vi "Device Files v1.vi"(10 "Rows":i32=80, 11 "Mask file path":path=path "C:/Documents and Settings/sjguest/Desktop/PVIV LV/Excel Files For Device Runs/All Devices.xls") -> (1 "Mask Name":string, 2 "size(s)":i32, 3 "Array of Cell Clusters":T2(array[cluster]), 4 "Alignment Spacing":cluster{"xintv":dbl, "yintv":dbl})   [LabVIEW 2012]
uses:
  <vilib>/imath/engines/lvmath2/RunTimeEngine/ErrorHandling/NIMS_Finalize Error.vi
  <vilib>/imath/engines/lvmath2/RunTimeEngine/NodeEndStatement/NIMS_NodeEndStatement_Output.vi
  <instcachedir>/0/NIMS_NodeEndStatement_Output_53EC0D466D134D7ABD903AC30B43404B.lvgen/NIMS_NodeEndStatement_Output_53EC0D466D134D7ABD903AC30B43404B_001.vi
  <vilib>/imath/engines/lvmath2/RunTimeEngine/BuiltInFunctions/sets_unique/NIMS_sets_unique(GV).vi
  <instcachedir>/0/NIMS_sets_unique(GV)_31CBCD1A87194FEB9DEFC0CB30627D6C.lvgen/NIMS_sets_unique(GV)_31CBCD1A87194FEB9DEFC0CB30627D6C_001.vi
  <vilib>/imath/engines/lvmath2/RunTimeEngine/BuiltInFunctions/length/NIMS_length(GV).vi
  <instcachedir>/0/NIMS_length(GV)_08A3D13377FD4E4B96F5795FBF3698FA.lvgen/NIMS_length(GV)_08A3D13377FD4E4B96F5795FBF3698FA_000.vi
  <vilib>/imath/engines/lvmath2/RunTimeEngine/BuiltInFunctions/abs/NIMS_abs(signed).vi
  <instcachedir>/0/NIMS_abs(signed)_C4FCB8E6058B49B797C7C8D53CA5F6EC.lvgen/NIMS_abs(signed)_C4FCB8E6058B49B797C7C8D53CA5F6EC_000.vi
  <vilib>/regexp/Match Regular Expression.xnode
panel:
  in  "Cell Info Cluster 2":T1={"Cell Name"="10000_150_06", "X-coord"=8850.0, "Y-coord"=8250.0, "Area"=99830016.0, "Grid Shadowing"=99830016.0, "Xdim"=99830016.0, "Ydim"=99830016.0, "Mesa Area"=0.0}
  out "yintv":dbl
  out "xintv":dbl
  out "data":dbl[][](array[numeric])
  out "Loop Count":i32
  out "selection":bool
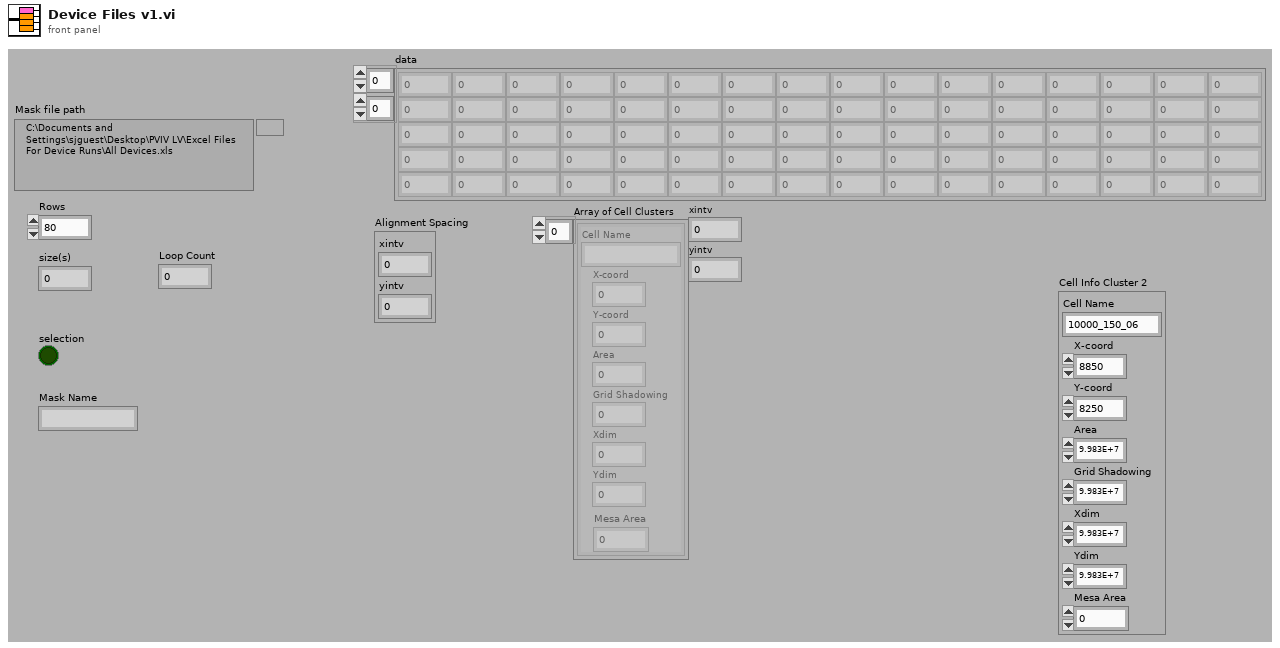
[diagram p1: front panel]
types:
  T1 = cluster{"Cell Name":string, "X-coord":dbl, "Y-coord":dbl, "Area":dbl, "Grid Shadowing":dbl, "Xdim":dbl, "Ydim":dbl, "Mesa Area":dbl}
  T2 = cluster{"Cell Name":string, "X-coord":dbl, "Y-coord":dbl, "Area":dbl, "Grid Shadowing":dbl, "Xdim":dbl, "Ydim":dbl, "Mesa Area":dbl}[]
  T3 = cluster{"disabled index (col)":i32, "disabled index (col)":i32}
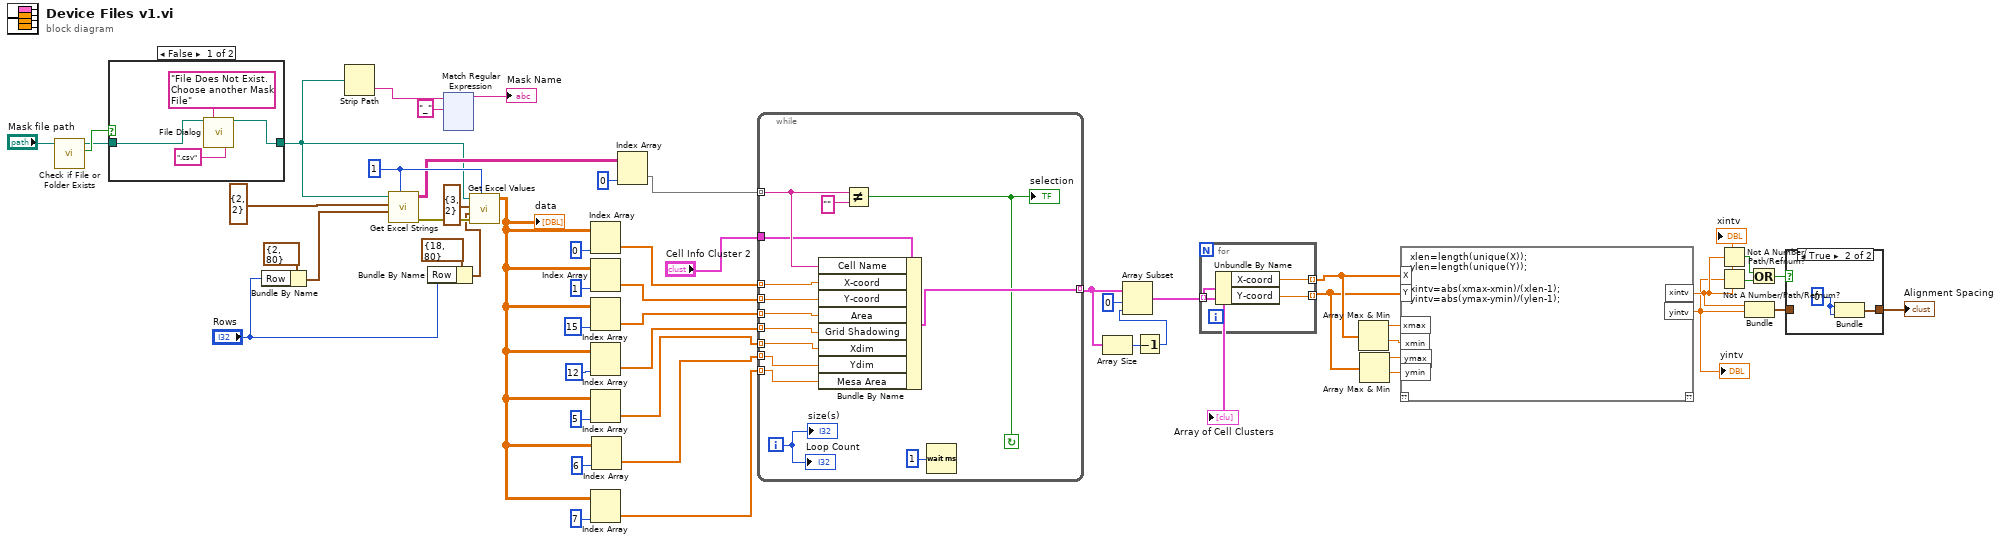
[diagram p0: block diagram]
diagram:
  w46 = 1 ("Sheet")
  n1 = call <vilib>:"Check if File or Folder Exists.vi"("path"="Mask file path") -> ("file or folder exists?"=w24:bool, "dup path"=w22:path)  [unwired: 8 in, 1 out]
  n2 = case shown="False" w24 {
    tunnel: [w56 w58] -> w23
    tunnel: w22 -> [w57 w58]
    frame False {
      n3 = call "File Dialog"("start path"=w57, "prompt"="File Does Not Exist.  Choose another Mask File", "pattern label"=".csv" ("pattern (all files)")) -> ("selected path"=w56:path)  [unwired: 9 in, 3 out]
    }
    frame True {
    }
  }
  n4 = Bundle By Name(cluster=cluster{"Column":i32, "Row":i32} {"Column"=2, "Row"=80} ("End"), "Row"="Rows") -> (w39:cluster{"Column":i32, "Row":i32})
  n5 = Strip Path(path=w23) -> (name=w28:string)  [unwired: 1 out]
  n6 = call "Get Excel Strings.vi"("Sheet"=w46, "End"=w39, "Start"=cluster{"Column":i32, "Row":i32} {"Column"=2, "Row"=2}, "path"=w23) -> ("error out"=w45:errorcluster, "data"=w42:string[][])  [unwired: 1 in, 5 out]
  n7 = Bundle By Name(cluster=cluster{"Column":i32, "Row":i32} {"Column"=18, "Row"=80} ("End"), "Row"="Rows") -> (w37:cluster{"Column":i32, "Row":i32})
  n8 = xnode "Match Regular Expression"("input string"=w28, "regular expression"="_") -> ("before match"=→"Mask Name":string)  [unwired: 2 in, 6 out]
  n9 = call "Get Excel Values.vi"("Sheet"=w46, "error in (no error)"=w45, "End"=w37, "Start"=cluster{"Column":i32, "Row":i32} {"Column"=3, "Row"=2}, "path"=w23) -> ("data"=w3:dbl[][])  [unwired: 6 out]
  "data" <- w3
  n10 = Index Array(array=w3, index (col)=0 ("disabled index (col)")) -> (element=w49:dbl[])  [unwired: 1 in]
  n11 = Index Array(array=w3, index (col)=1 ("disabled index (col)")) -> (element=w48:dbl[])  [unwired: 1 in]
  n12 = Index Array(array=w3, index (col)=15 ("disabled index (col)")) -> (element=w47:dbl[])  [unwired: 1 in]
  n13 = Index Array(array=w3, index (col)=12 ("disabled index (col)")) -> (element=w33:dbl[])  [unwired: 1 in]
  n14 = Index Array(array=w3, index (col)=5 ("disabled index (col)")) -> (element=w12:dbl[])  [unwired: 1 in]
  n15 = Index Array(array=w3, index (col)=7 ("disabled index (col)")) -> (element=w2:dbl[])  [unwired: 1 in]
  n16 = Index Array(array=w3, index (col)=6 ("disabled index (col)")) -> (element=w11:dbl[])  [unwired: 1 in]
  n17 = Index Array(array=w42, index (col)=0 ("disabled index (col)")) -> (element=w53:string[])  [unwired: 1 in]
  n18 = while {
    tunnel: w53 -> [w67] mode=indexing
    tunnel: w49 -> [w70] mode=indexing
    tunnel: w48 -> [w69] mode=indexing
    tunnel: w47 -> [w68] mode=indexing
    tunnel: "Cell Info Cluster 2" -> [w66]
    tunnel: [w64] -> w25 mode=indexing
    tunnel: w33 -> [w65] mode=indexing
    tunnel: w12 -> [w61] mode=indexing
    tunnel: w11 -> [w60] mode=indexing
    tunnel: w2 -> [w59] mode=indexing
    i -> [w62]
    stop <- w63 continue-if-true
    n19 = Bundle By Name(cluster=w66, "Cell Name"=w67, "X-coord"=w70, "Y-coord"=w69, "Area"=w68, "Grid Shadowing"=w65, "Xdim"=w61, "Ydim"=w60, "Mesa Area"=w59) -> (w64:T1)
    n20 = Not Equal?(x=w67, y="" ("false string")) -> (x != y?=w63:bool)
    "selection" <- w63
    n21 = Wait (ms)(milliseconds to wait=u32 1) -> ()  [unwired: 1 out]
    "Loop Count" <- w62
    "size(s)" <- w62
  }
  n22 = Array Size(array=w25) -> (size(s)=w31:i32)
  n23 = Decrement(x=w31) -> (x-1=w30:i32)
  n24 = Array Subset(array=w25, index=0, length=w30) -> (w21:T2)
  "Array of Cell Clusters" <- w21
  n25 = for {
    tunnel: w21 -> [w75] mode=indexing
    tunnel: [w74] -> w20 mode=indexing
    tunnel: [w73] -> w19 mode=indexing
    n26 = Unbundle By Name(w75) -> ("X-coord"=w74:dbl, "Y-coord"=w73:dbl)
  }
  n27 = Array Max & Min(array=w20) -> (max value=w15:dbl, min value=w16:dbl)  [unwired: 2 out]
  n28 = Array Max & Min(array=w19) -> (max value=w17:dbl, min value=w18:dbl)  [unwired: 2 out]
  n29 = mathscript code="xlen=length(unique(X));\nylen=length(unique(Y));\n\nxintv=abs(xmax-xmin)/(xlen-1);\nyintv=abs(ymax-ymin)/(ylen-1);"("X"=w20, "Y"=w19, "xmax"=w15, "xmin"=w16, "ymax"=w17, "ymin"=w18) -> ("xintv"=w10:dbl, "yintv"=w9:dbl)  [unwired: 1 in, 1 out]
  "xintv" <- w10
  "yintv" <- w9
  n30 = Not A Number/Path/Refnum?(number/path/refnum=w10) -> (NaN/Path/Refnum?=w8:bool)
  n31 = Not A Number/Path/Refnum?(number/path/refnum=w9) -> (NaN/Path/Refnum?=w7:bool)
  n32 = Bundle("xintv"=w10, "yintv"=w9) -> (w5:cluster{"xintv":dbl, "yintv":dbl})  [unwired: 1 in]
  n33 = Or(x=w8, y=w7) -> (x .or. y?=w6:bool)
  n34 = case shown="True" w6 {
    tunnel: w5 -> [w76 _]
    tunnel: [w76 w78] -> w4
    frame False {
    }
    frame True {
      w77 = 0 ("disabled index (col)")
      n35 = Bundle("disabled index (col)"=w77, "disabled index (col)"=w77) -> (w78:T3)  [unwired: 1 in]
    }
  }
  "Alignment Spacing" <- w4
